vi "Result_Test.vi"(8 "error in (no error)":errorcluster caption="entrée d'erreur (pas d'erreur)", 11 "Get_Voltage en entrée":refnum<class "Zigbee_Send_Command_UART.lvclass">) -> (0 "error out":errorcluster caption="sortie d'erreur", 3 "Get_Voltage en sortie":refnum<class "Zigbee_Send_Command_UART.lvclass">)   [LabVIEW 2020, in "Library Test.lvlib" / "Zigbee_Send_Command_UART.lvclass"]
uses:
  Zigbee_Send_Command_UART.lvclass
  Commun VI/TypeDef/Variable Printable.ctl
  Test_Wtih_Instr/Test_With_Inst.lvclass
  Commun VI/Library Commun.lvlib
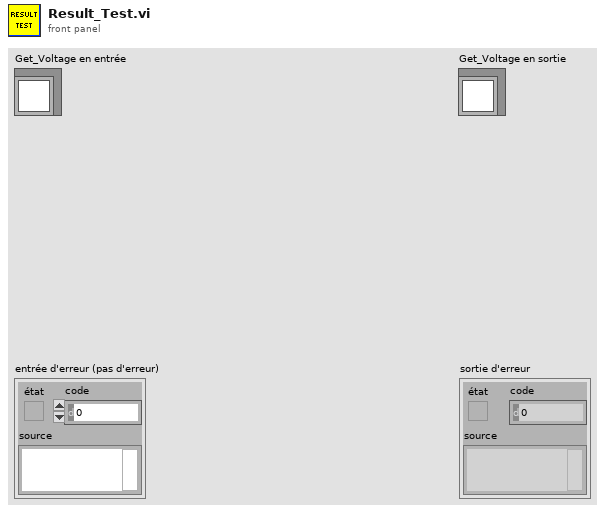
[diagram p1: front panel]
types:
  T1 = typedef "Variable Printable.ctl" = string
  T2 = enum16{"Get Variable", "Get All Variables", "Set Variable", "Delete Variable", "Delete All Variable"}
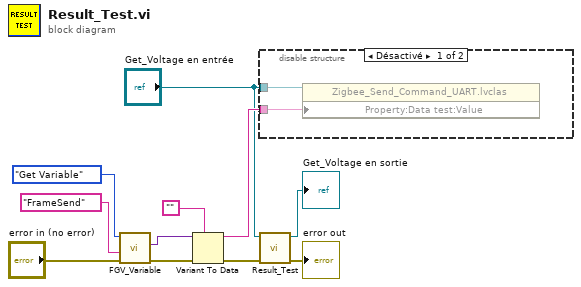
[diagram p0: block diagram]
diagram:
  n1 = call "FGV_Variable.vi"("error in (no error)"="error in (no error)", "Variable"=T1 "FrameSend", "Function"=T2."Get Variable") -> ("error out"=w4:errorcluster, "Data Out"=w6:variant)  [unwired: 6 in, 1 out]
  n2 = Variant To Data(error in=w4, type="", Variant=w6) -> (data=w5:string, error out=w1:errorcluster)
  n3 = disable-structure shown="Désactivé" {
    disable-tunnel: w5 -> [w13 _]
    disable-tunnel: "Get_Voltage en entrée" -> [w12 _]
    frame Disabled {
      n4 = property class="Zigbee_Send_Command_UART.lvclas"(reference=w12, "Property:Data test:Value"=w13) -> ()  [unwired: 1 in, 2 out]
    }
    frame Enabled {
    }
  }
  n5 = call-parent "Result_Test.vi"("error in (no error)"=w1, "Test_With_Inst en entrée"="Get_Voltage en entrée") -> ("error out"=→"error out":errorcluster, "Test_With_Inst en sortie"=→"Get_Voltage en sortie":refnum<class "Zigbee_Send_Command_UART.lvclass">)  [unwired: 8 in]
